vi "Compare Folders.vi"(8 "error in (no error)":errorcluster, 10 "Folder 2":path, 11 "Folder 1":path) -> (0 "error out":errorcluster)   [LabVIEW 2014, in "SLL File IO.lvlib"]
doc: "Compare two folders and provide the list of \n1. Files Modified\n2. Files Deleted\n3. Files Added\n\nThis uses CRC check to validate if the files have been modiied or not."
uses:
  SLL File IO.lvlib
panel:
  in  "Folders to Exclude":string[](array[string])
  out "Files Deleted":path[](array[path])
  out "Files Added":path[](array[path])
  out "Files Modified":path[](array[path])
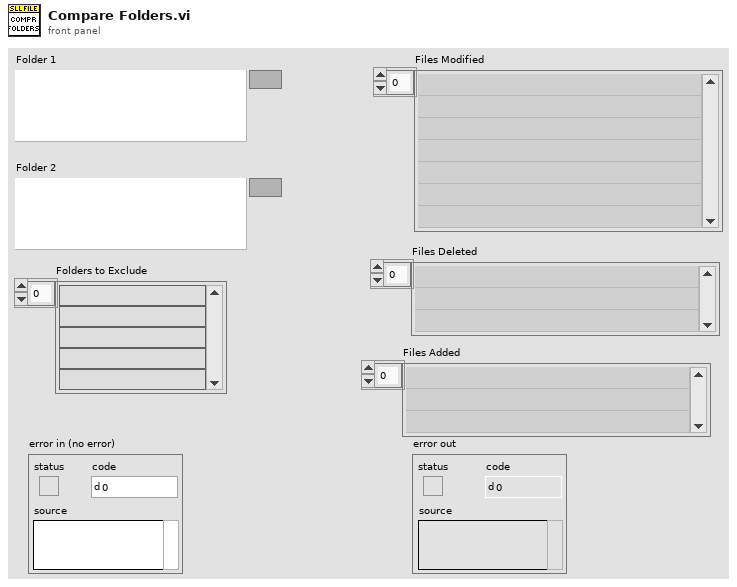
[diagram p1: front panel]
types:
  T1 = typedef "SLL File IO.lvlib/Folder Shot Element.ctl" = cluster{"Abs.Path":path, "Relative Path":path, "MD5":string}
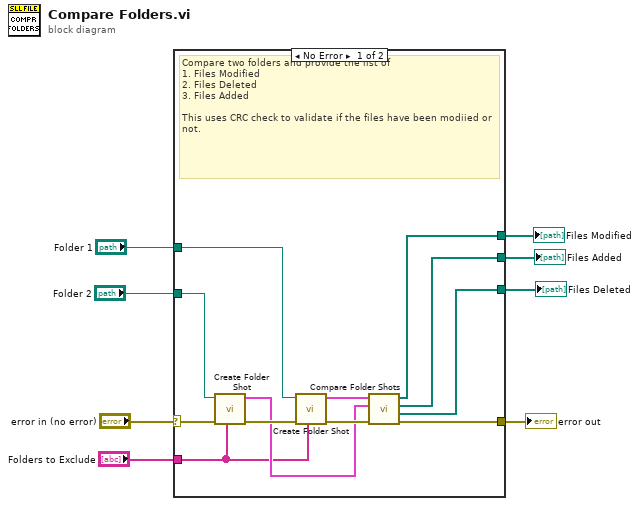
[diagram p0: block diagram]
diagram:
  n1 = case shown="No Error" "error in (no error)" {
    selector: "error in (no error)" -> [w20 w21]
    tunnel: [w15 w21] -> w7
    tunnel: "Folder 2" -> [w18 _]
    tunnel: "Folder 1" -> [w16 _]
    tunnel: [w12 _] -> w4
    tunnel: [w11 _] -> w3
    tunnel: [w10 _] -> w2
    tunnel: "Folders to Exclude" -> [w9 _]
    frame No Error {
      # "Compare two folders and provide the list of \n1. Files Modified\n2. Files Deleted\n3. Files Added\n\nThis uses CRC check to validate if the files have been modiied or not."
      n2 = call "Create Folder Shot.vi"("Folders to Exclude"=w9, "error in (no error)"=w20, "Directory Path"=w18) -> ("error out"=w19:errorcluster, "Folder Shot"=w13:T1[])  [unwired: 7 in]
      n3 = call "Create Folder Shot.vi"("Folders to Exclude"=w9, "error in (no error)"=w19, "Directory Path"=w16) -> ("error out"=w17:errorcluster, "Folder Shot"=w14:T1[])  [unwired: 7 in]
      n4 = call "Compare Folder Shots.vi"("error in (no error)"=w17, "Folder Shot 2"=w13, "Folder Shot 1"=w14) -> ("error out"=w15:errorcluster, "Files Deleted"=w10:path[], "Files Added"=w11:path[], "Files Modified"=w12:path[])  [unwired: 5 in]
    }
    frame Error {
    }
  }
  "error out" <- w7
  "Files Modified" <- w4
  "Files Added" <- w3
  "Files Deleted" <- w2
